vi "Control.vi"(4 "dt":dbl, 6 "t[s]":dbl, 7 "CIVITA Euler Angles DMARS seq [rad]":cluster{"phi":dbl, "theta":dbl, "psi":dbl}, 8 "all rows":dbl[][](array[numeric]), 9 "M_ab":dbl[](array[numeric]), 10 "q (i+1)":dbl[](array[numeric]), 11 "V(i) (m/s)":dbl[](array[numeric])) -> (0 "yaw P out(i)[deg]":dbl, 1 "yaw ref [deg]":dbl, 2 "pitch ref [deg]":dbl, 3 "TVA_cmd(i+1,:) [rad]":dbl[](array[numeric]))   [LabVIEW 2017]
uses:
  <vilib>/Analysis/coordinate.llb/Euler Rotation Order.ctl
  <vilib>/Analysis/_algsub.llb/Vector Norm Type.ctl
  <vilib>/Analysis/_algsub.llb/Real Vector Norm.vi
  <vilib>/Analysis/NI_AALPro.lvlib
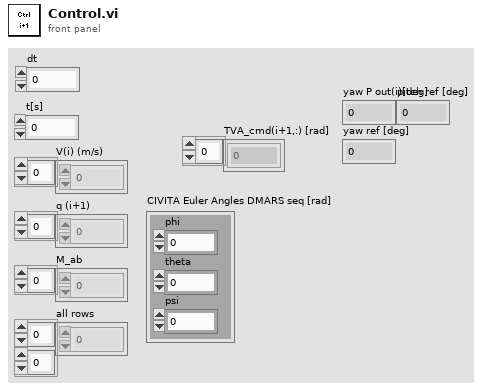
[diagram p1: front panel]
types:
  T1 = typedef "NI_AALPro.lvlib/Vector Norm Type.ctl" = u16
  T2 = typedef "NI_AALPro.lvlib/Euler Rotation Order.ctl" = u16
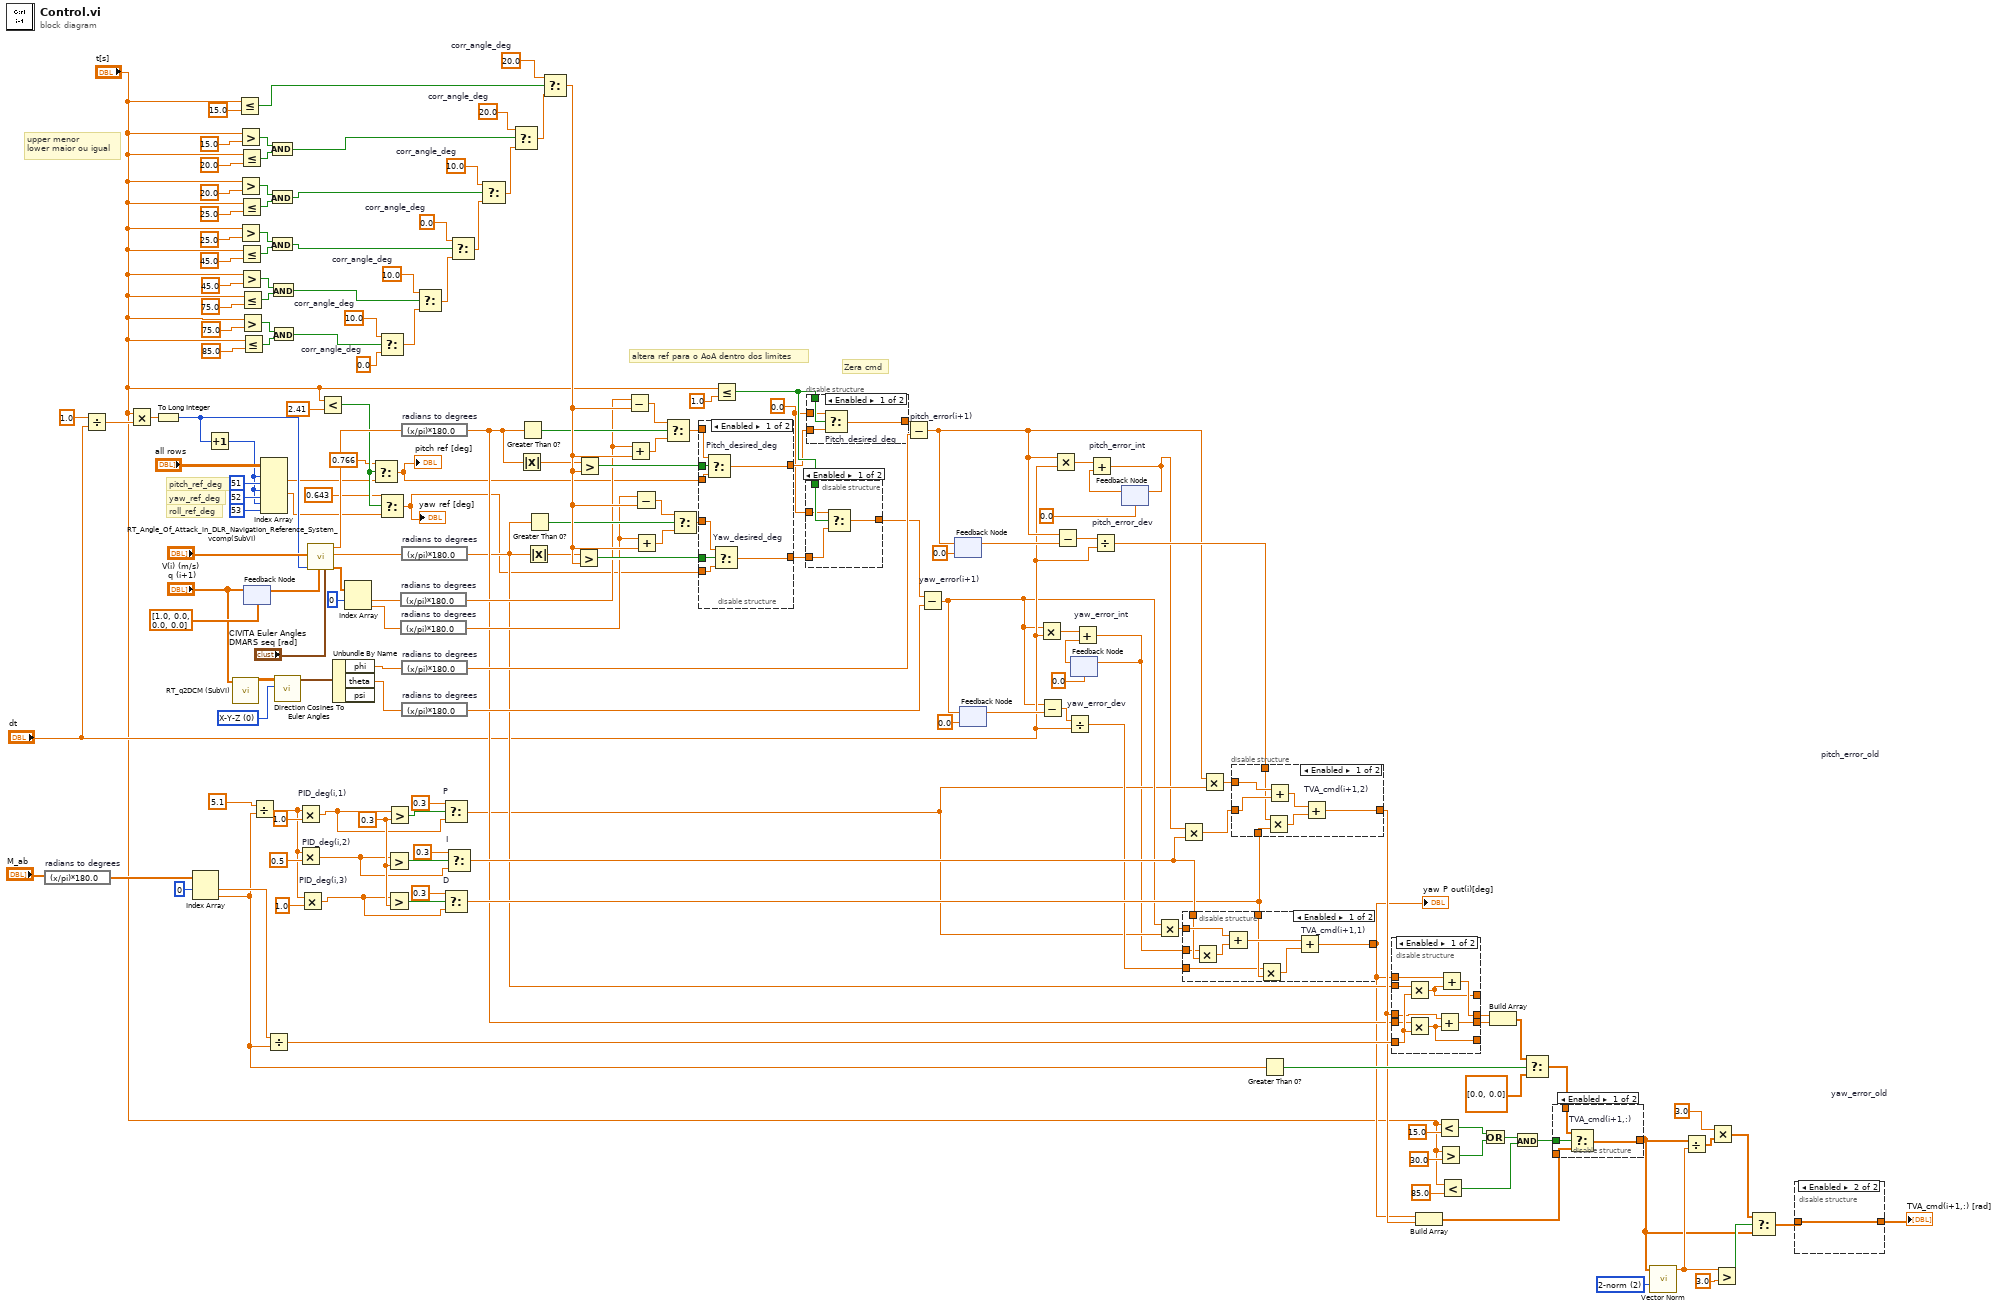
[diagram p0: block diagram]
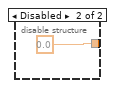
[diagram p2: hidden frame]
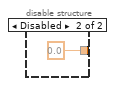
[diagram p7: hidden frame]
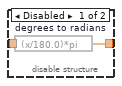
[diagram p9: hidden frame]
diagram:
  w42 = 0.0 ("t")
  w66 = T1 2 items=["1-norm"=1, "2-norm"=2, "Inf-norm"=3, "-Inf-norm"=4, "User Defined"=5] ("norm type")
  w100 = 0.3 ("y")
  w120 = T2 0 items=["X-Y-Z", "X-Z-Y", "Y-X-Z", "Y-Z-X", "Z-X-Y", "Z-Y-X", "X-Y-X", "X-Z-X", "Y-X-Y", "Y-Z-Y", "Z-X-Z", "Z-Y-Z"] ("rotation order")
  w134 = 0.0  # corr_angle_deg
  w137 = 10.0  # corr_angle_deg
  w140 = 10.0  # corr_angle_deg
  w165 = 0.0  # corr_angle_deg
  w167 = 10.0  # corr_angle_deg
  w169 = 20.0  # corr_angle_deg
  w170 = 20.0  # corr_angle_deg
  # "Zera cmd"
  # "altera ref para o AoA dentro dos limites"
  # "roll_ref_deg"
  # "yaw_ref_deg"
  # "pitch_ref_deg"
  # "upper menor\nlower maior ou igual"
  n1 = expression code="(x/pi)*180.0" "radians to degrees"("M_ab") -> (w71:dbl[])
  n2 = Divide(x=1.0, y="dt") -> (x/y=w24:dbl)
  n3 = Multiply(x="t[s]", y=w24) -> (x*y=w132:dbl)
  n4 = To Long Integer(number=w132) -> (32bit integer=w115:i32)
  n5 = Index Array(array=w71, index #1=0 ("index")) -> (element #1=w70:dbl, element #2=w69:dbl)  [unwired: 1 in]
  n6 = Increment(x=w115) -> (x+1=w114:i32)
  n7 = call "RT_q2DCM (SubVI).vi"("Quaternion"="q (i+1)") -> ("DCM"=w121:dbl[][])  [unwired: 10 in]
  n8 = Less Or Equal?(x="t[s]", y=15.0) -> (x <= y?=w171:bool)
  n9 = Greater?(x="t[s]", y=15.0) -> (0:w161:bool)
  n10 = Greater?(x="t[s]", y=20.0) -> (0:w157:bool)
  n11 = Greater?(x="t[s]", y=25.0) -> (0:w152:bool)
  n12 = Less Or Equal?(x="t[s]", y=20.0) -> (x <= y?=w160:bool)
  n13 = Less Or Equal?(x="t[s]", y=25.0) -> (x <= y?=w158:bool)
  n14 = Less Or Equal?(x="t[s]", y=45.0) -> (x <= y?=w151:bool)
  n15 = Greater?(x="t[s]", y=45.0) -> (0:w149:bool)
  n16 = Less Or Equal?(x="t[s]", y=75.0) -> (x <= y?=w150:bool)
  n17 = Greater?(x="t[s]", y=75.0) -> (0:w144:bool)
  n18 = Less Or Equal?(x="t[s]", y=85.0) -> (x <= y?=w143:bool)
  n19 = feedback-in #1("q (i+1)") -> ()
  n20 = feedback #1(dbl[] [1.0, 0.0, 0.0, 0.0] ("q (i+1)")) -> (w117:dbl[])
  n21 = Divide(x=5.1, y=w69) -> (x/y=w101:dbl)
  n22 = Index Array(array="all rows", index (row) #1=w114, index (col) #1=51 ("disabled index (col)"), index (row) #2=w114, index (col) #2=52 ("disabled index (col)"), index (row) #3=w114, index (col) #3=53 ("disabled index (col)")) -> (element #1=w4:dbl, element #2=w3:dbl)  [unwired: 1 out]
  n23 = Divide(x=w70, y=w69) -> (x/y=w68:dbl)
  n24 = And(x=w161, y=w160) -> (x .and. y?=w159:bool)
  n25 = And(x=w157, y=w158) -> (x .and. y?=w142:bool)
  n26 = And(x=w152, y=w151) -> (x .and. y?=w141:bool)
  n27 = And(x=w149, y=w150) -> (x .and. y?=w139:bool)
  n28 = And(x=w144, y=w143) -> (x .and. y?=w136:bool)
  n29 = call <vilib>:"Direction Cosines To Euler Angles.vi"("rotation order"=w120, "Direction Cosines"=w121) -> ("Euler Angles"=w10:cluster{"phi":dbl, "theta":dbl, "psi":dbl})  [unwired: 8 in, 1 out]
  n30 = Multiply "PID_deg(i,1)"(x=w101, y=1.0) -> (x*y=w97:dbl)
  n31 = Multiply "PID_deg(i,2)"(x=w101, y=0.5) -> (x*y=w92:dbl)
  n32 = Multiply "PID_deg(i,3)"(x=w101, y=1.0) -> (x*y=w91:dbl)
  n33 = call "RT_Angle_Of_Attack_in_DLR_Navigation_Reference_System_vcomp(SubVI).vi"("Euler Angles [rad]"="CIVITA Euler Angles DMARS seq [rad]", "q"=w117, "i"=w115, "V (m/s)"="V(i) (m/s)") -> ("Speed_direction [rad]"=w125:dbl[], "AoA_yaw (rad)"=w122:dbl, "AoA_pitch (rad)"=w32:dbl)  [unwired: 5 in]
  n34 = Less?(x="t[s]", y=2.41) -> (x < y?=w5:bool)
  n35 = Unbundle By Name(w10) -> ("phi"=w119:dbl, "theta"=w118:dbl)  [unwired: 1 out]
  n36 = Index Array(array=w125, index #1=0 ("index")) -> (element #1=w126:dbl, element #2=w127:dbl)  [unwired: 1 in]
  n37 = Select(t=0.766, s=w5, f=w4) -> (s? t:f=w9:dbl)
  "pitch ref [deg]" <- w9
  n38 = Select(t=w137, s=w136, f=w134) -> (s? t:f=w135:dbl)
  n39 = Select(t=0.643, s=w5, f=w3) -> (s? t:f=w8:dbl)
  "yaw ref [deg]" <- w8
  n40 = Greater?(x=w92, y=w100) -> (0:w93:bool)
  n41 = Greater?(x=w91, y=w100) -> (0:w94:bool)
  n42 = Greater?(x=w97, y=w100) -> (0:w99:bool)
  n43 = expression code="(x/pi)*180.0" "radians to degrees"(w126) -> (w30:dbl)
  n44 = expression code="(x/pi)*180.0" "radians to degrees"(w127) -> (w31:dbl)
  n45 = expression code="(x/pi)*180.0" "radians to degrees"(w32) -> (w28:dbl)
  n46 = expression code="(x/pi)*180.0" "radians to degrees"(w122) -> (w25:dbl)
  n47 = expression code="(x/pi)*180.0" "radians to degrees"(w119) -> (w112:dbl)
  n48 = expression code="(x/pi)*180.0" "radians to degrees"(w118) -> (w106:dbl)
  n49 = Select(t=w140, s=w139, f=w135) -> (s? t:f=w138:dbl)
  n50 = Select "P"(t=0.3, s=w99, f=w97) -> (s? t:f=w18:dbl)
  n51 = Select "D"(t=0.3, s=w94, f=w91) -> (s? t:f=w86:dbl)
  n52 = Select "I"(t=0.3, s=w93, f=w92) -> (s? t:f=w87:dbl)
  n53 = Select(t=w165, s=w141, f=w138) -> (s? t:f=w164:dbl)
  n54 = Select(t=w167, s=w142, f=w164) -> (s? t:f=w166:dbl)
  n55 = Select(t=w169, s=w159, f=w166) -> (s? t:f=w168:dbl)
  n56 = Absolute Value(x=w28) -> (abs(x)=w58:dbl)
  n57 = Greater Than 0?(x=w28) -> (x > 0?=w55:bool)
  n58 = Absolute Value(x=w25) -> (abs(x)=w47:dbl)
  n59 = Greater Than 0?(x=w25) -> (x > 0?=w50:bool)
  n60 = Select(t=w170, s=w171, f=w168) -> (s? t:f=w123:dbl)
  n61 = Greater?(x=w47, y=w123) -> (0:w48:bool)
  n62 = Greater?(x=w58, y=w123) -> (0:w57:bool)
  n63 = Subtract(x=w30, y=w123) -> (x-y=w54:dbl)
  n64 = Add(x=w30, y=w123) -> (x+y=w53:dbl)
  n65 = Subtract(x=w31, y=w123) -> (x-y=w51:dbl)
  n66 = Add(x=w31, y=w123) -> (x+y=w52:dbl)
  n67 = Select(t=w54, s=w55, f=w53) -> (s? t:f=w56:dbl)
  n68 = Select(t=w51, s=w50, f=w52) -> (s? t:f=w49:dbl)
  n69 = disable-structure shown="Enabled" {
    disable-tunnel: w8 -> [w180 w181]
    disable-tunnel: w9 -> [w179 w182]
    disable-tunnel: w57 -> [w178 _]
    disable-tunnel: w56 -> [w177 _]
    disable-tunnel: w49 -> [w176 _]
    disable-tunnel: w48 -> [w175 _]
    disable-tunnel: [w174 w182] -> w44
    disable-tunnel: [w173 w181] -> w43
    frame Enabled {
      n70 = Select "Pitch_desired_deg"(t=w177, s=w178, f=w179) -> (s? t:f=w174:dbl)
      n71 = Select "Yaw_desired_deg"(t=w176, s=w175, f=w180) -> (s? t:f=w173:dbl)
    }
    frame Disabled {
    }
  }
  n72 = Less Or Equal?(x="t[s]", y=1.0) -> (x <= y?=w45:bool)
  n73 = disable-structure shown="Enabled" {
    disable-tunnel: [w186 0.0 ("t")] -> w19
    disable-tunnel: w45 -> [w185 _]
    disable-tunnel: w43 -> [w184 _]
    disable-tunnel: w42 -> [w183 _]
    frame Enabled {
      n74 = Select ("Yaw_desired_deg")(t=w183, s=w185, f=w184) -> (s? t:f=w186:dbl)
    }
    frame Disabled {
    }
  }
  n75 = disable-structure shown="Enabled" {
    disable-tunnel: [w191 0.0 ("t")] -> w113
    disable-tunnel: w45 -> [w190 _]
    disable-tunnel: w44 -> [w189 _]
    disable-tunnel: w42 -> [w188 _]
    frame Enabled {
      n76 = Select "Pitch_desired_deg"(t=w188, s=w190, f=w189) -> (s? t:f=w191:dbl)
    }
    frame Disabled {
    }
  }
  n77 = Subtract "pitch_error(i+1)"(x=w113, y=w112) -> (x-y=w35:dbl)
  n78 = Subtract "yaw_error(i+1)"(x=w19, y=w106) -> (x-y=w20:dbl)
  n79 = feedback #2 "pitch_error_old"(0.0) -> (w41:dbl)
  n80 = feedback-in #2(w35) -> ()
  n81 = feedback #3 "yaw_error_old"(0.0) -> (w39:dbl)
  n82 = feedback-in #3(w20) -> ()
  n83 = Multiply(x=w20, y="dt") -> (x*y=w109:dbl)
  n84 = Subtract ("yaw_error_dev")(x=w20, y=w39) -> (x-y=w38:dbl)
  n85 = Multiply(x=w35, y="dt") -> (x*y=w16:dbl)
  n86 = Subtract ("pitch_error_dev")(x=w35, y=w41) -> (x-y=w40:dbl)
  n87 = Divide "yaw_error_dev"(x=w38, y="dt") -> (x/y=w37:dbl)
  n88 = feedback #4(0.0) -> (w107:dbl)
  n89 = Add "yaw_error_int"(x=w109, y=w107) -> (x+y=w12:dbl)
  n90 = feedback-in #4(w12) -> ()
  n91 = Divide "pitch_error_dev"(x=w40, y="dt") -> (x/y=w36:dbl)
  n92 = feedback #5(0.0) -> (w15:dbl)
  n93 = Add "pitch_error_int"(x=w16, y=w15) -> (x+y=w13:dbl)
  n94 = feedback-in #5(w13) -> ()
  n95 = Multiply(x=w20, y=w18) -> (x*y=w88:dbl)
  n96 = Multiply(x=w13, y=w87) -> (x*y=w89:dbl)
  n97 = disable-structure shown="Enabled" {
    disable-tunnel: w88 -> [w198 w202]
    disable-tunnel: w87 -> [w197 _]
    disable-tunnel: w86 -> [w196 _]
    disable-tunnel: w12 -> [w195 _]
    disable-tunnel: w37 -> [w194 _]
    disable-tunnel: [w193 w202] -> w17
    frame Enabled {
      n98 = Multiply(x=w195, y=w197) -> (x*y=w199:dbl)
      n99 = Add(x=w198, y=w199) -> (x+y=w200:dbl)
      n100 = Multiply(x=w194, y=w196) -> (x*y=w201:dbl)
      n101 = Add "TVA_cmd(i+1,1)"(x=w200, y=w201) -> (x+y=w193:dbl)
    }
    frame Disabled {
    }
  }
  "yaw P out(i)[deg]" <- w17
  n102 = Multiply(x=w35, y=w18) -> (x*y=w90:dbl)
  n103 = disable-structure shown="Enabled" {
    disable-tunnel: w90 -> [w209 w210]
    disable-tunnel: w89 -> [w208 _]
    disable-tunnel: w86 -> [w205 _]
    disable-tunnel: [w204 w210] -> w29
    disable-tunnel: w36 -> [w203 _]
    frame Enabled {
      n104 = Multiply(x=w203, y=w205) -> (x*y=w206:dbl)
      n105 = Add(x=w209, y=w208) -> (x+y=w207:dbl)
      n106 = Add "TVA_cmd(i+1,2)"(x=w207, y=w206) -> (x+y=w204:dbl)
    }
    frame Disabled {
    }
  }
  n107 = Greater Than 0?(x=w69) -> (x > 0?=w75:bool)
  n108 = disable-structure shown="Enabled" {
    disable-tunnel: w68 -> [w219 _]
    disable-tunnel: w25 -> [w218 _]
    disable-tunnel: w28 -> [w217 _]
    disable-tunnel: w17 -> [w216 w220]
    disable-tunnel: w29 -> [w214 w221]
    disable-tunnel: [w215 w220] -> w27
    disable-tunnel: [w213 w221] -> w26
    disable-tunnel: [w212 _] -> _
    disable-tunnel: [w211 _] -> _
    frame Enabled {
      n109 = Multiply(x=w218, y=w219) -> (x*y=w212:dbl)
      n110 = Multiply(x=w217, y=w219) -> (x*y=w211:dbl)
      n111 = Add(x=w214, y=w211) -> (x+y=w213:dbl)
      n112 = Add(x=w216, y=w212) -> (x+y=w215:dbl)
    }
    frame Disabled {
    }
  }
  n113 = Build Array(w17, w29) -> (w76:dbl[])
  n114 = Less?(x="t[s]", y=15.0) -> (x < y?=w85:bool)
  n115 = Greater?(x="t[s]", y=30.0) -> (0:w83:bool)
  n116 = Less?(x="t[s]", y=85.0) -> (x < y?=w79:bool)
  n117 = Or(x=w85, y=w83) -> (x .or. y?=w80:bool)
  n118 = Build Array(w27, w26) -> (w67:dbl[])
  n119 = And(x=w80, y=w79) -> (x .and. y?=w78:bool)
  n120 = Select(t=w67, s=w75, f=dbl[] [0.0, 0.0] ("appended array")) -> (s? t:f=w77:dbl[])
  n121 = disable-structure shown="Enabled" {
    disable-tunnel: w78 -> [w225 _]
    disable-tunnel: w77 -> [w224 _]
    disable-tunnel: w76 -> [w223 w226]
    disable-tunnel: [w222 w226] -> w34
    frame Enabled {
      n122 = Select "TVA_cmd(i+1,:)"(t=w224, s=w225, f=w223) -> (s? t:f=w222:dbl[])
    }
    frame Disabled {
    }
  }
  n123 = call-poly <vilib>:"Vector Norm.vi"("norm type"=w66, "Input Vector"=w34) -> ("norm"=w63:dbl)  [unwired: 8 in, 1 out]
  n124 = Divide(x=w34, y=w63) -> (x/y=w61:dbl[])
  n125 = Multiply(x=3.0, y=w61) -> (x*y=w60:dbl[])
  n126 = Greater?(x=w63, y=3.0) -> (0:w64:bool)
  n127 = Select(t=w60, s=w64, f=w34) -> (s? t:f=w33:dbl[])
  n128 = disable-structure shown="Enabled" {
    disable-tunnel: w33 -> [w228 w229]
    disable-tunnel: [w227 w229] -> w59
    frame Disabled {
      n129 = expression code="(x/180.0)*pi" "degrees to radians"(w228) -> (w227:dbl[])
    }
    frame Enabled {
    }
  }
  "TVA_cmd(i+1,:) [rad]" <- w59
